vi "To Bulleted String.vi"(11 "projpath error message":string) -> (3 "string":string)   [LabVIEW 2013, in "DecideModuleFeatures.lvclass"]
uses:
  DecideModuleFeatures.lvclass
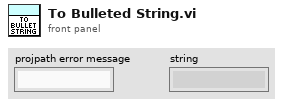
[diagram p1: front panel]
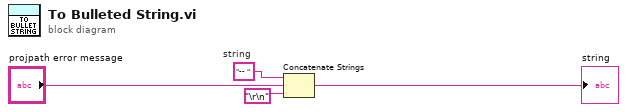
[diagram p0: block diagram]
diagram:
  w2 = "-- "  # string
  n1 = Concatenate Strings(w2, "projpath error message", "\r\n") -> (→"string":string)
